vi "CheckIfPropertyExist.vi"(8 "error in (no error)":errorcluster, 9 "ClusterOfProperties":refnum<vi>, 10 "properties":T1) -> (0 "error out":errorcluster, 1 "ClusterOfProperties":refnum<vi>, 2 "Exists":bool, 4 "TypeMatches":bool)   [LabVIEW 2013, in "GenLVOOP.lvclass"]
uses:
  GenLVOOP.lvclass
  baseClass/propertyDef.ctl
  baseClass/types.ctl
  baseClass/baseClass.lvclass
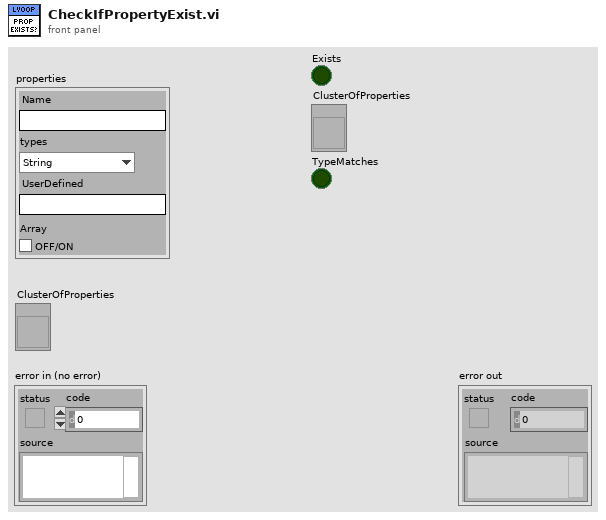
[diagram p1: front panel]
types:
  T1 = typedef "baseClass.lvclass/propertyDef.ctl" = cluster{"Name":string, "types":T2, "UserDefined":string, "Array":bool}
  T2 = typedef "baseClass.lvclass/types.ctl" = enum16{"String", "Int32", "Uint32", "Array", "Class", "Double", "Enum"}
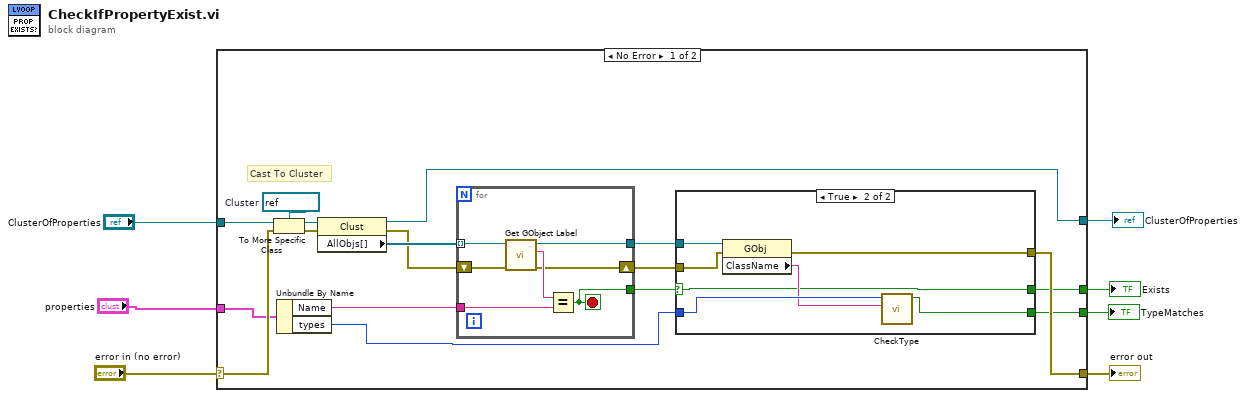
[diagram p0: block diagram]
diagram:
  n1 = case shown="No Error" "error in (no error)" {
    selector: "error in (no error)" -> [w19 w41]
    tunnel: [w11 w41] -> w6
    tunnel: "ClusterOfProperties" -> [w18 _]
    tunnel: [w17 _] -> w4
    tunnel: "properties" -> [w16 _]
    tunnel: [w10 _] -> w2
    tunnel: [w8 _] -> w1
    frame No Error {
      w24 = refnum<vi> refnum  # Cluster
      # "Cast To Cluster"
      n2 = To More Specific Class(target class=w24, reference=w18, error in=w19) -> (specific class reference=w22:refnum<vi>, error out=w23:errorcluster)
      n3 = Unbundle By Name(w16) -> ("Name"=w15:string, "types"=w9:T2)
      n4 = property class="Clust"(reference=w22, error in=w23) -> (reference out=w17:refnum<vi>, error out=w20:errorcluster, "AllObjs[]"=w21:refnum<vi>[])
      n5 = for {
        tunnel: w21 -> [w40] mode=indexing
        tunnel: w15 -> [w38]
        tunnel: [w37] -> w14
        shift-right: [w36] -> w13
        shift-left: w20 -> [w35]
        tunnel: [w34] -> w12
        stop <- w37 stop-if-true
        n6 = call <vilib>:"Get GObject Label.vi"("error in (no error)"=w35, "GObject"=w40) -> ("error out"=w36:errorcluster, "Object Label"=w39:string, "dup GObject"=w34:refnum<vi>)  [unwired: 5 in, 2 out]
        n7 = Equal?(x=w39, y=w38) -> (x = y?=w37:bool)
      }
      n8 = case shown="True" w14 {
        selector: w14 -> [w25 w28]
        tunnel: w13 -> [w26 w33]
        tunnel: w12 -> [_ w32]
        tunnel: [w26 w31] -> w11
        tunnel: [w25 w28] -> w10
        tunnel: w9 -> [_ w30]
        tunnel: [_ w27] -> w8
        frame False {
        }
        frame True {
          n9 = property class="GObj"(reference=w32, error in=w33) -> (error out=w31:errorcluster, "ClassName"=w29:string)  [unwired: 1 out]
          n10 = call "CheckType.vi"("Class Name"=w29, "types"=w30) -> ("TypeMatch"=w27:bool)  [unwired: 9 in]
        }
      }
    }
    frame Error {
    }
  }
  "error out" <- w6
  "Exists" <- w2
  "ClusterOfProperties" <- w4
  "TypeMatches" <- w1
